vi "Write Transfer Groups.vi"(8 "error in (no error)":errorcluster, 10 "Transfer Groups":refnum<class "Configuration.Transfer Group.lvclass">[](array[class]), 11 "Plugin Configuration in":refnum<class "Plugin Configuration.lvclass">) -> (0 "error out":errorcluster, 3 "Plugin Configuration out":refnum<class "Plugin Configuration.lvclass">)   [LabVIEW 2016, in "Plugin Configuration.lvclass"]
uses:
  Plugin Configuration.lvclass
  Configuration.Transfer Group/Configuration.Transfer Group.lvclass
  Plugin Configuration.lvclass/Plugin Configuration.ctl
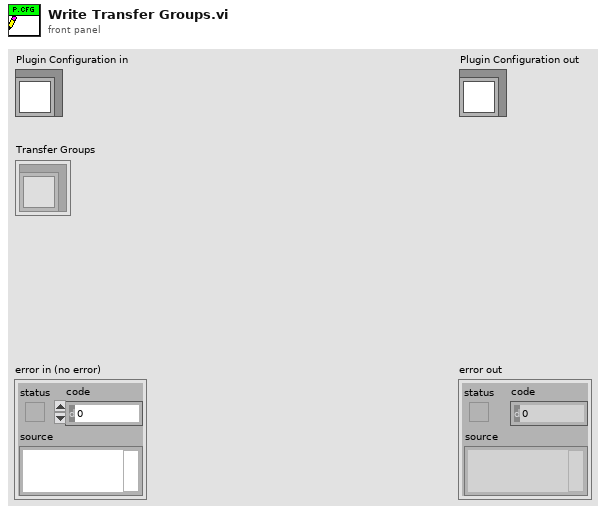
[diagram p1: front panel]
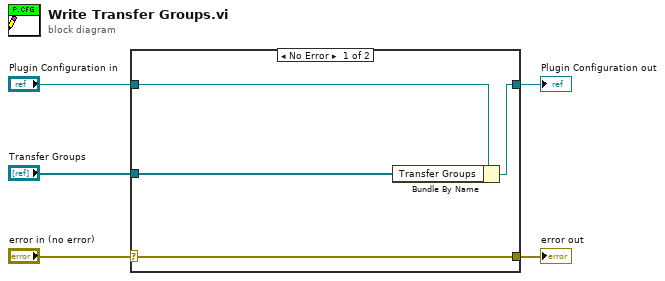
[diagram p0: block diagram]
diagram:
  n1 = case shown="No Error" "error in (no error)" {
    selector: "error in (no error)" -> [w9 w10]
    tunnel: [w9 w10] -> w4
    tunnel: [w7 w11] -> w2
    tunnel: "Plugin Configuration in" -> [w8 w11]
    tunnel: "Transfer Groups" -> [w6 _]
    frame No Error {
      n2 = Bundle By Name(cluster=w8, "Transfer Groups"=w6) -> (w7:refnum<class "Plugin Configuration.lvclass">)
    }
    frame Error {
    }
  }
  "error out" <- w4
  "Plugin Configuration out" <- w2
